vi "SetPosition(degree).vi"(8 "error in (no error)":errorcluster, 10 "degree":dbl, 11 "Motor Base in":refnum<class "Motor Base.lvclass">) -> (0 "error out":errorcluster, 3 "Motor Base out":refnum<class "Motor Base.lvclass">)   [LabVIEW 2016, in "Motor Base.lvlib" / "Motor Base.lvclass"]
uses:
  Motor Base.lvclass
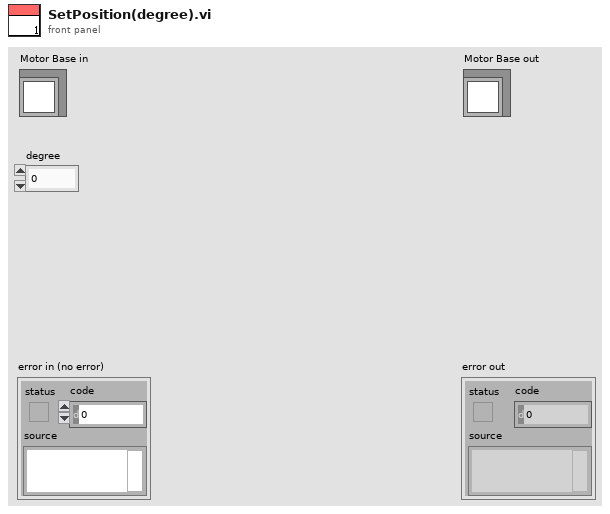
[diagram p1: front panel]
types:
  T1 = cluster{"Modes of operation":i8, "Feed(pulse)":u32, "Max motor speed(r/min)":u32, "Max torque(0.1%)":u16, "Min position limit(pulse)":i32, "Max position limit(pulse)":i32}
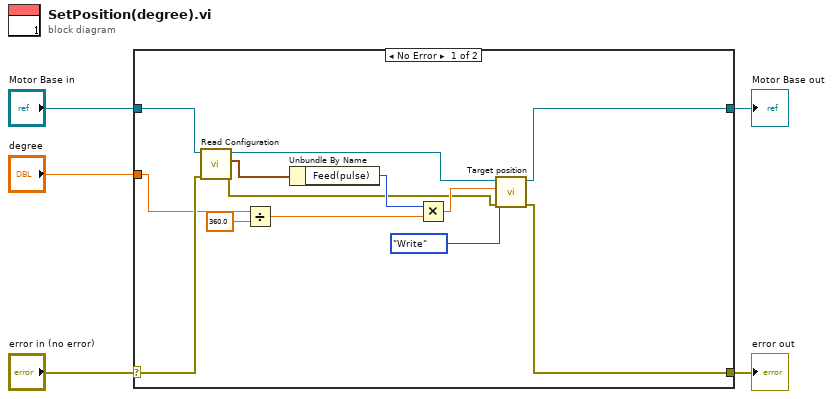
[diagram p0: block diagram]
diagram:
  n1 = case shown="No Error" "error in (no error)" {
    selector: "error in (no error)" -> [w17 w20]
    tunnel: [w8 w20] -> w4
    tunnel: [w7 w19] -> w2
    tunnel: "Motor Base in" -> [w18 w19]
    tunnel: "degree" -> [w15 _]
    frame No Error {
      n2 = call-dynamic "Read Configuration.vi"("error in (no error)"=w17, "Motor Base in"=w18) -> ("error out"=w9:errorcluster, "Configuration"=w16:T1, "Motor Base out"=w11:refnum<class "Motor Base.lvclass">)  [unwired: 7 in]
      n3 = Divide(x=w15, y=360.0) -> (x/y=w12:dbl)
      n4 = Unbundle By Name(w16) -> ("Feed(pulse)"=w13:u32)
      n5 = Multiply(x=w13, y=w12) -> (x*y=w10:dbl)
      n6 = call-dynamic "Target position.vi"("error in"=w9, "W/R"=enum16{"Write", "Read"}."Write", "Data"=w10, "Motor Base in"=w11) -> ("error out"=w8:errorcluster, "Motor Base out"=w7:refnum<class "Motor Base.lvclass">)  [unwired: 5 in, 1 out]
    }
    frame Error {
    }
  }
  "error out" <- w4
  "Motor Base out" <- w2
